vi "Numeric Control (Silver).vi"() -> ()   [LabVIEW 2012]
panel:
  in  "Numeric Control":dbl
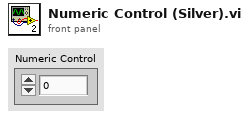
[diagram p1: front panel]
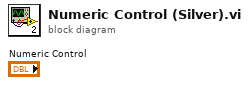
[diagram p0: block diagram]
diagram:
